vi "Blood pressure realtime.vi"() -> ()   [LabVIEW 2019]
uses:
  <vilib>/Analysis/3filter.llb/Filter Passband Type.ctl
  <vilib>/DAQmx/read.llb/DAQmx Read (Analog DBL 1Chan 1Samp).vi
  <vilib>/DAQmx/create/channels.llb/DAQmx Create Channel (AI-Voltage-Basic).vi
  <vilib>/DAQmx/configure/timing.llb/DAQmx Timing (Sample Clock).vi
  <vilib>/DAQmx/miscellaneous.llb/DAQmx Fill In Error Info.vi
  <vilib>/Analysis/3filter.llb/Butterworth Filter (DBL).vi
  <vilib>/Analysis/NI_AALBase.lvlib
panel:
  out "Max value":dbl
  out "Index of Max":dbl
  out "Maximum after Gate":dbl
  out "MAP":dbl[](array[numeric])
  out "XY Graph":cluster{"Array":dbl[], "Filtered X":dbl[]}(graph)
  out "Sampling frequency":dbl
  out "Filtered sig":dbl[](graph)
  out "Total Samples":dbl
  out "Cuff pressure":dbl
  out "Pressure graph":dynamicdata(graph)
  in  "Clear chart":bool
  out "Window of Pressure graph":dynamicdata(graph)
  out "Real time Pressure":dbl(graph)
  in  "Stop":bool
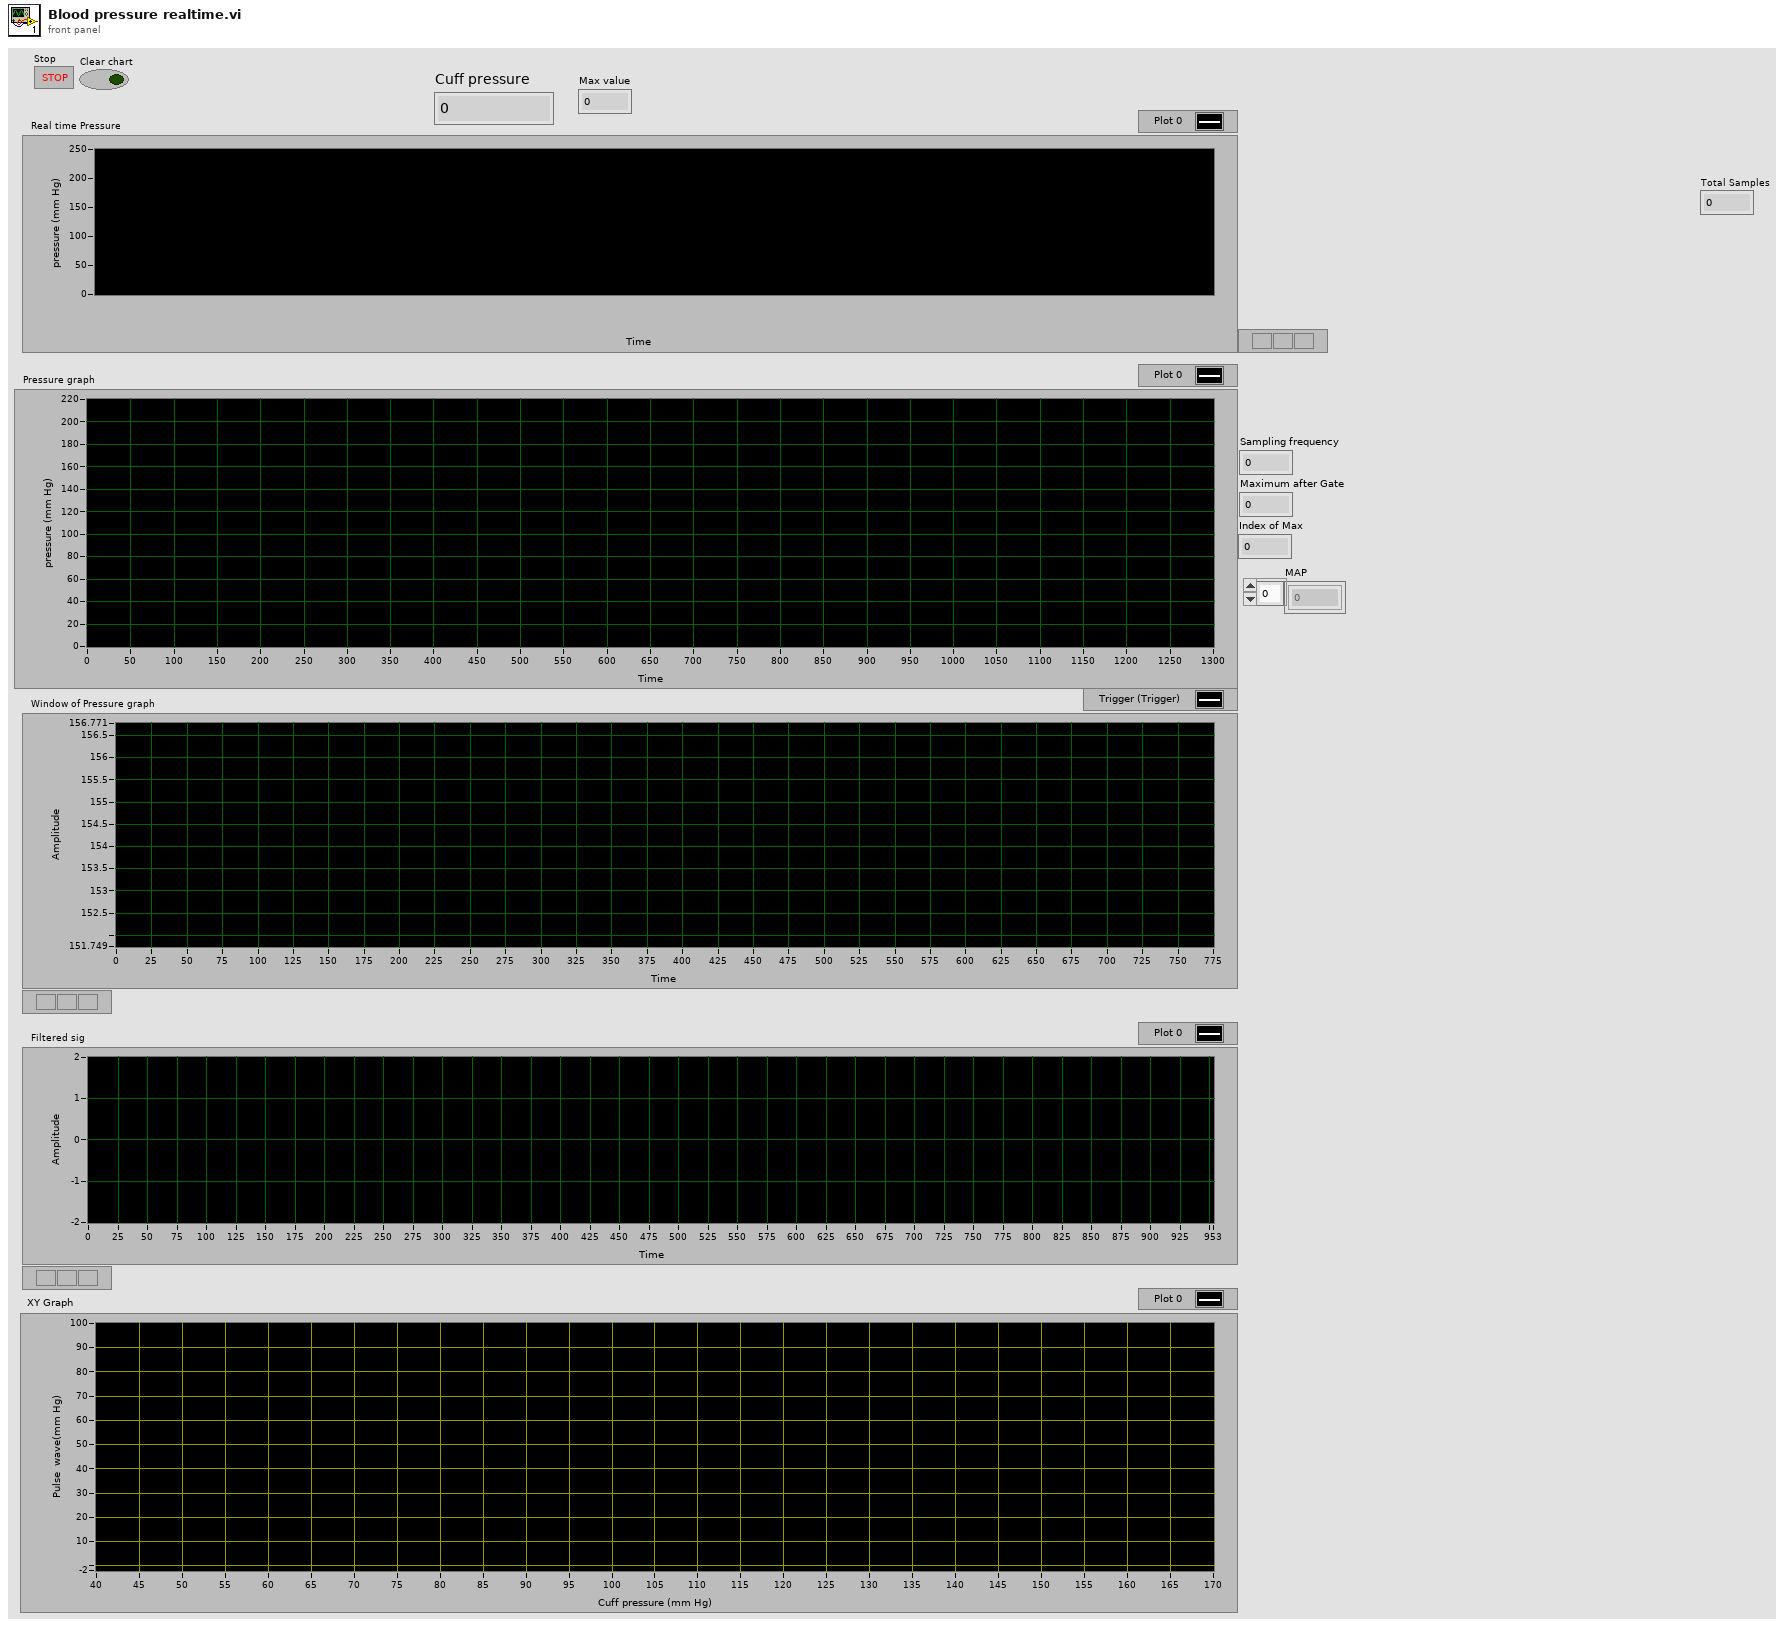
[diagram p1: front panel]
types:
  T1 = typedef "NI_AALBase.lvlib/Filter Passband Type.ctl" = enum32{"Lowpass", "Highpass", "Bandpass", "Bandstop"}
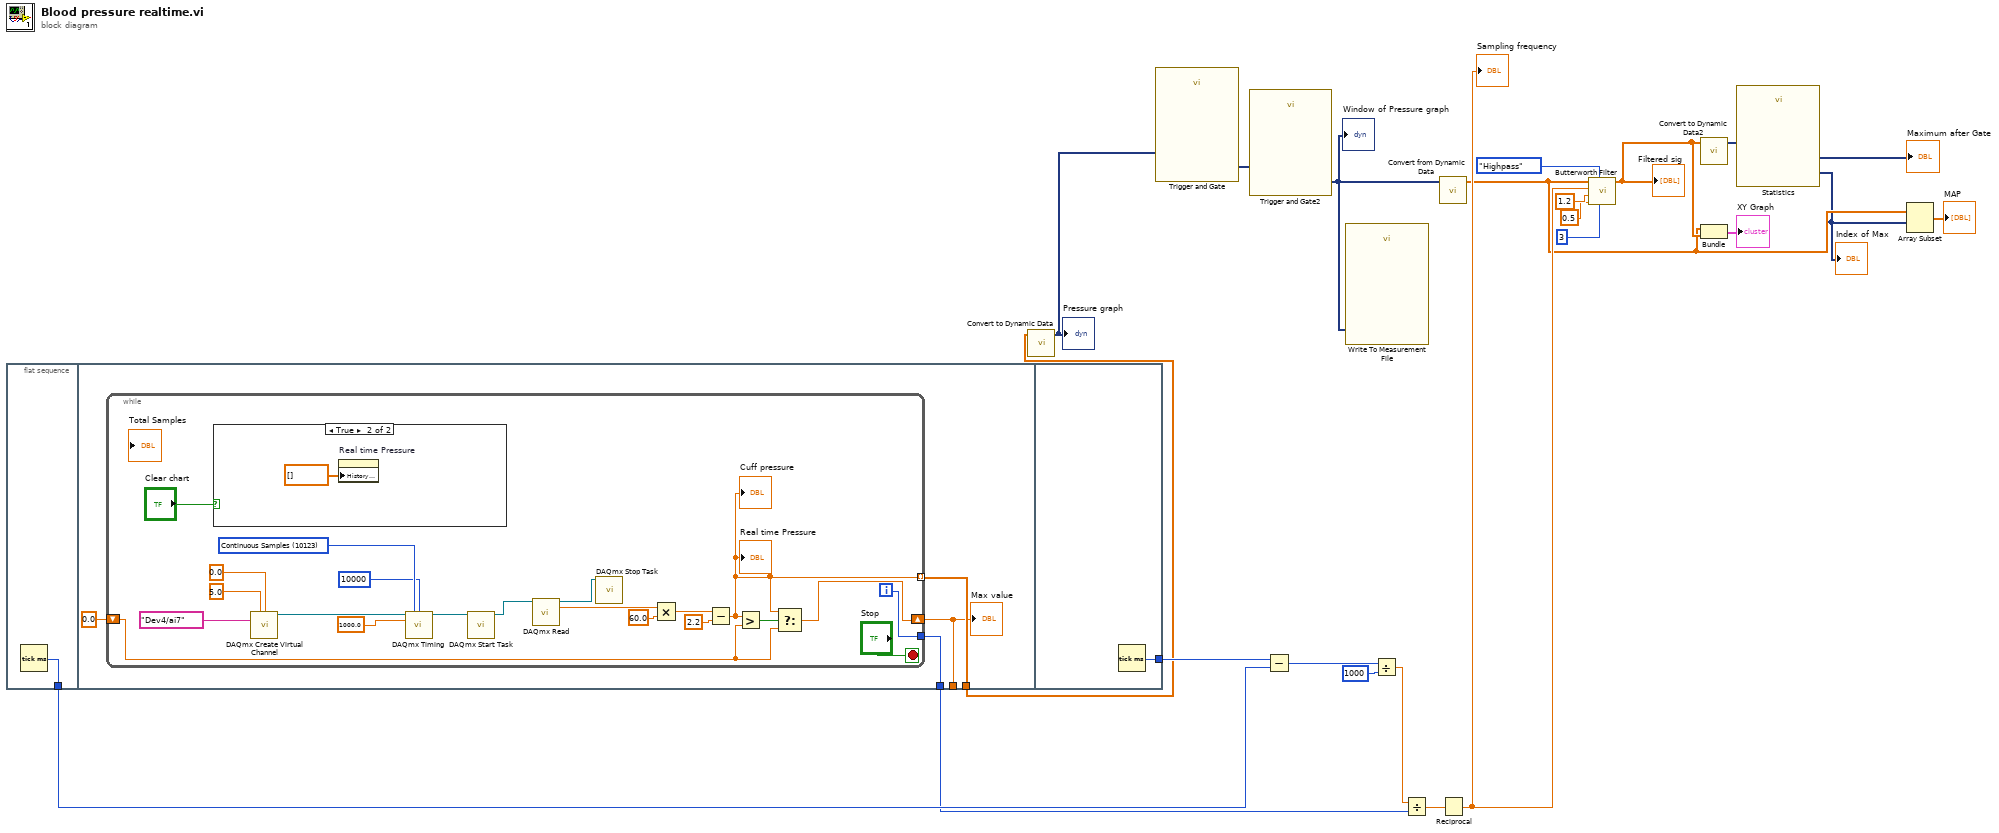
[diagram p0: block diagram]
diagram:
  n1 = flat-sequence {
    tunnel: [w24] -> w19
    tunnel: [w28] -> w3
    tunnel: [w27] -> w15
    tunnel: [w25] -> _
    tunnel: [w51] -> w20
    frame #0 {
      n2 = Tick Count (ms)() -> (millisecond timer value=w24:u32)
    }
    frame #1 {
      n3 = while {
        tunnel: [w30] -> w28 mode=indexing
        tunnel: [w33] -> w27
        shift-right: [w32] -> w25
        shift-left: 0.0 -> [w31]
        i -> [w33]
        stop <- "Stop" stop-if-true
        w45 = 10123 items=["Finite Samples"=10178, "Continuous Samples"=10123, "Hardware Timed Single Point"=12522] ("sample mode")
        n4 = case shown="True" "Clear chart" {
          frame False {
          }
          frame True {
            n5 = property on="Real time Pressure" class="WFChart (strict)"("History Data"=dbl[] []) -> ()  [unwired: 2 in, 2 out]
          }
        }
        n6 = call-poly <vilib>:"DAQmx Create Virtual Channel.vi"("maximum value"=5.0, "minimum value"=0.0, "physical channels"=tag "Dev4/ai7") -> ("task out"=w46:refnum<k21>)  [unwired: 11 in, 1 out]
        n7 = call-poly <vilib>:"DAQmx Timing.vi"("task/channels in"=w46, "sample mode"=w45, "samples per channel"=10000, "rate"=1000.0) -> ("task out"=w42:refnum<k21>)  [unwired: 10 in, 1 out]
        n8 = call <vilib>:"DAQmx Start Task.vi"("task/channels in"=w42) -> ("task out"=w41:refnum<k21>)  [unwired: 13 in, 1 out]
        n9 = call-poly <vilib>:"DAQmx Read.vi"("task/channels in"=w41) -> ("task out"=w40:refnum<k21>, "data"=w38:dbl)  [unwired: 12 in, 1 out]
        n10 = call <vilib>:"DAQmx Stop Task.vi"("task/channels in"=w40) -> ()  [unwired: 13 in, 2 out]
        n11 = Multiply(x=w38, y=60.0) -> (x*y=w37:dbl)
        n12 = Subtract(x=w37, y=2.2) -> (x-y=w30:dbl)
        "Real time Pressure" <- w30
        "Cuff pressure" <- w30
        n13 = Greater?(x=w30, y=w31) -> (0:w29:bool)
        n14 = Select(t=w30, s=w29, f=w31) -> (s? t:f=w32:dbl)
      }
      "Max value" <- w25
    }
    frame #2 {
      n15 = Tick Count (ms)() -> (millisecond timer value=w51:u32)
    }
  }
  n16 = call "Convert to Dynamic Data"("Array"=w3) -> ("Dynamic Data Type"=w21:dynamicdata)  [unwired: 3 in]
  "Pressure graph" <- w21
  n17 = call "Trigger and Gate"("Signals"=w21) -> ("Triggered Signals"=w2:dynamicdata)  [unwired: 7 in, 3 out]
  n18 = call "Trigger and Gate2"("Signals"=w2) -> ("Triggered Signals"=w1:dynamicdata)  [unwired: 7 in, 3 out]
  "Window of Pressure graph" <- w1
  n19 = Subtract(x=w20, y=w19) -> (x-y=w18:u32)
  n20 = call "Write To Measurement File"("Signals"=w1) -> ()  [unwired: 16 in, 3 out]
  n21 = Divide(x=w18, y=u32 1000) -> (x/y=w16:dbl)
  n22 = Divide(x=w16, y=w15) -> (x/y=w14:dbl)
  n23 = call "Convert from Dynamic Data"("Dynamic Data Type"=w1) -> ("Array"=w7:dbl[])  [unwired: 3 in]
  n24 = Reciprocal(x=w14) -> (1/x=w13:dbl)
  "Sampling frequency" <- w13
  n25 = call-poly <vilib>:"Butterworth Filter.vi"("order"=3, "filter type"=Filter_Passband_Type."Highpass", "low cutoff freq: fl"=0.5, "high cutoff freq: fh"=1.2, "sampling freq: fs"=w13, "X"=w7) -> ("Filtered X"=w9:dbl[])  [unwired: 2 in, 1 out]
  "Filtered sig" <- w9
  n26 = call "Convert to Dynamic Data2"("Array"=w9) -> ("Dynamic Data Type"=w8:dynamicdata)  [unwired: 3 in]
  n27 = Bundle("Array"=w7, "Filtered X"=w9) -> (→"XY Graph":cluster{"Array":dbl[], "Filtered X":dbl[]})  [unwired: 1 in]
  n28 = call "Statistics"("Signals"=w8) -> ("Index of Max"=w6:dynamicdata, "Maximum"=→"Maximum after Gate":dynamicdata)  [unwired: 24 in, 1 out]
  "Index of Max" <- w6
  n29 = Array Subset(array=w7, index=w6) -> (→"MAP":dbl[])  [unwired: 1 in]
